vi "type_44_timestamp_two_channels_one_segment.vi"() -> ()   [LabVIEW 2010]
panel:
  out "error out":errorcluster
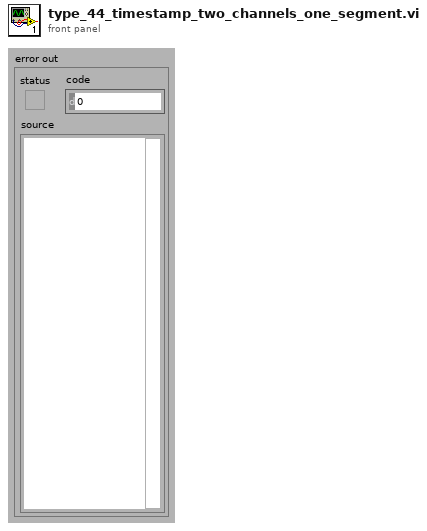
[diagram p1: front panel]
types:
  T1 = enum16{"open", "open or create", "create or replace", "create", "open (read-only)"}
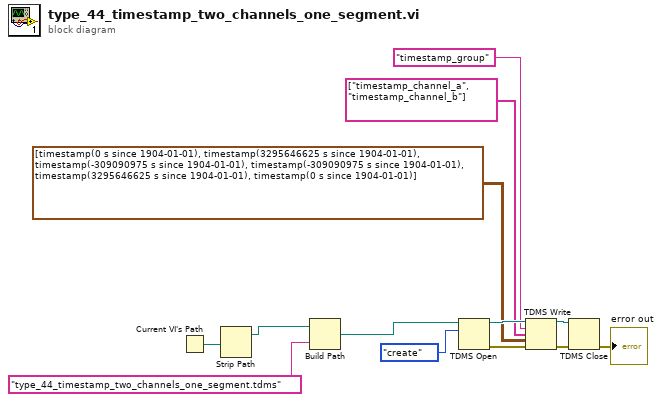
[diagram p0: block diagram]
diagram:
  n1 = Current VI's Path() -> (path=w6:path)
  n2 = Strip Path(path=w6) -> (stripped path=w5:path)  [unwired: 1 out]
  n3 = Build Path(base path=w5, name or relative path="type_44_timestamp_two_channels_one_segment.tdms") -> (appended path=w3:path)
  n4 = TDMS Open(10:T1."create" ("operation (0:open)"), 11:w3) -> (0:w13:errorcluster, 3:w12:refnum<k34>)  [unwired: 4 in]
  n5 = TDMS Write(0:w12, 5:"timestamp_group" ("group name in (Untitled)"), 7:string[] ["timestamp_channel_a", "timestamp_channel_b"] ("channel name(s) in (Untitled)"), 9:timestamp[][] [[timestamp(0 s since 1904-01-01), timestamp(3295646625 s since 1904-01-01), timestamp(-309090975 s since 1904-01-01)], [timestamp(-309090975 s since 1904-01-01), timestamp(3295646625 s since 1904-01-01), timestamp(0 s since 1904-01-01)]], 11:w13) -> (4:w9:refnum<k34>, 15:w8:errorcluster)  [unwired: 1 in, 2 out]
  n6 = TDMS Close(8:w8, 11:w9) -> (0:→"error out":errorcluster)  [unwired: 1 out]
